vi "IRTransmissionlogref av elec140617_SD.vi"(1 "Moyenne par pas":i8=4, 2 "resultat_input":dbl[](array[numeric])=array[24576 elements]) -> (0 "Résultat DO":dbl[][](array[numeric]))   [LabVIEW 2015]
panel:
  # "Transmission: on fait le log après la moyenne.\n\nCe VI comporte une entrée Dark: dark shutter fermé. La laisser à 0 \nce dark doit être retiré à toute les données, puis on doit faire le meme calcul avec le reste de Idark -dark à la place de Idark.s"
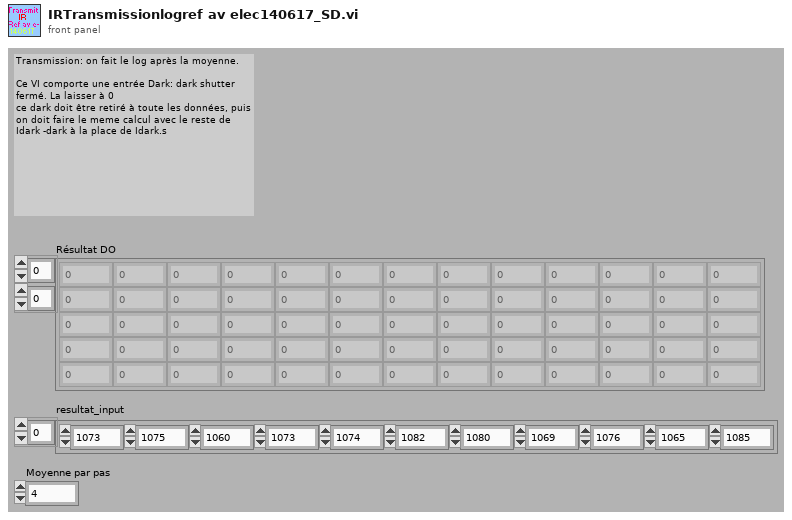
[diagram p1: front panel]
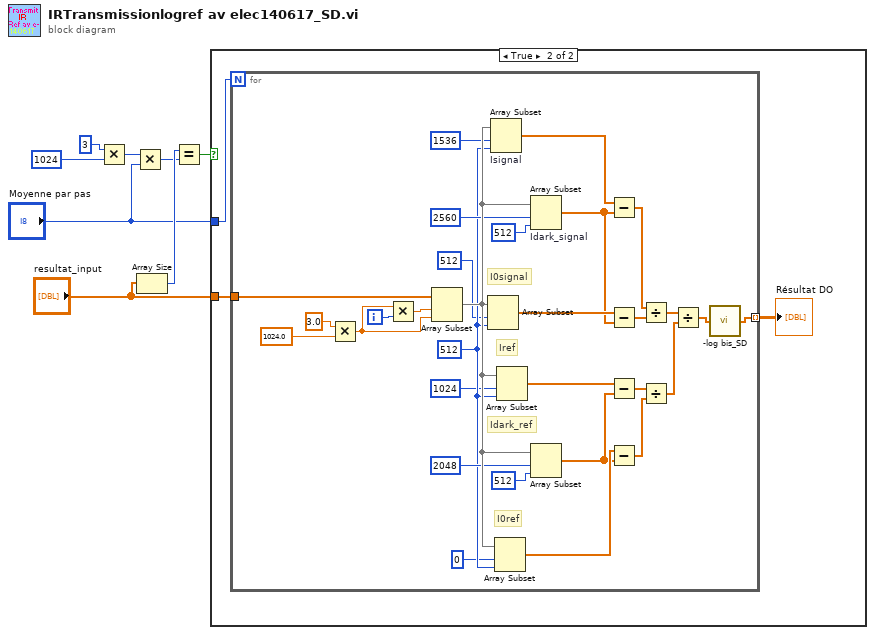
[diagram p0: block diagram]
diagram:
  n1 = Multiply(x=3, y=1024) -> (x*y=w6:i32)
  n2 = Multiply(x=w6, y="Moyenne par pas") -> (x*y=w4:i32)
  n3 = Array Size(array="resultat_input") -> (size(s)=w5:i32)
  n4 = Equal?(x=w5, y=w4) -> (x = y?=w3:bool)
  n5 = case shown="True" w3 {
    tunnel: "resultat_input" -> [_ w11]
    tunnel: "Moyenne par pas" -> [_ w10]
    frame False {
    }
    frame True {
      n6 = for {
        N: w10 -> [_]
        tunnel: w11 -> [w39]
        tunnel: [w12] -> w9 mode=indexing
        i -> [w21]
        w18 = 512 ("longueur")
        # "Idark_ref"
        # "I0signal"
        # "I0ref"
        # "Iref"
        n7 = Multiply(x=3.0, y=1024.0) -> (x*y=w37:dbl)
        n8 = Multiply(x=w37, y=w21) -> (x*y=w38:dbl)
        n9 = Array Subset(array=w39, index=w38, length=w37) -> (w26:dbl[])
        n10 = Array Subset(array=w26, index=512 ("indice"), length=w18) -> (w33:dbl[])
        n11 = Array Subset "Isignal"(array=w26, index=1536 ("indice"), length=w18) -> (w35:dbl[])
        n12 = Array Subset(array=w26, index=0 ("indice"), length=w18) -> (w34:dbl[])
        n13 = Array Subset(array=w26, index=1024 ("indice"), length=w18) -> (w36:dbl[])
        n14 = Array Subset "Idark_signal"(array=w26, index=2560 ("indice"), length=512 ("longueur")) -> (w19:dbl[])
        n15 = Array Subset(array=w26, index=2048 ("indice"), length=512 ("longueur")) -> (w20:dbl[])
        n16 = Subtract(x=w35, y=w19) -> (x-y=w32:dbl[])
        n17 = Subtract(x=w33, y=w19) -> (x-y=w31:dbl[])
        n18 = Subtract(x=w36, y=w20) -> (x-y=w30:dbl[])
        n19 = Subtract(x=w34, y=w20) -> (x-y=w29:dbl[])
        n20 = Divide(x=w32, y=w31) -> (x/y=w28:dbl[])
        n21 = Divide(x=w30, y=w29) -> (x/y=w27:dbl[])
        n22 = Divide(x=w28, y=w27) -> (x/y=w13:dbl[])
        n23 = call "-log bis_SD.vi"("Transmission"=w13) -> ("-log(x)=log(1/x)"=w12:dbl[])
      }
      "Résultat DO" <- w9
    }
  }
